vi "Main 2.vi"() -> ()   [LabVIEW 2017, in "HostCode.lvlib"]
doc: "This VI was generated automatically using the FPGA Wizard. You can modify the VI normally."
uses:
  HostCode.lvlib
  FPGACode/Lead Enum.ctl
  Trigger Params.ctl
  FPGACode/Channel Enum.ctl
  <vilib>/FPGAPlugInAG/Dynamic/niLvFpga_Reset_Dynamic.vi
  <vilib>/FPGAPlugInAG/Dynamic/niLvFpga_Run_Dynamic.vi
  <vilib>/Utility/error.llb/Error Cluster From Error Code.vi
  <vilib>/rvi/errors/niLvFpgaAdjustHostInterfaceError.vi
  <vilib>/FPGAPlugInAG/Dynamic/niLvFpga_Close_Dynamic.vi
  <vilib>/rvi/interface/nirviMethod/nirviMethod.xnode
  <vilib>/rvi/interface/nirviReadWriteControl/nirviReadWriteControl.xnode
  <vilib>/rvi/interface/nirviCloseFPGA/nirviCloseFPGA.xnode
  <vilib>/rvi/interface/Simulation/niFpgaSimulationCallBeginRW.vi
  <vilib>/FPGAPlugInAG/Dynamic/niLvFpga_ReadFifo_Dynamic.vi
  <vilib>/rvi/errors/niLvFpgaMergeErrorWithErrorCode.vi
  NiFpgaLv.dll
panel:
  in  "Beta":u8(slide)=1 scale=0.0..3.0
  in  "Sensis\nECG Scaling":i16=1 caption="ECG Output\nScaling" min=1 max=100 step=1
  in  "Tab Control":enum32{"Main", "Utilities"}(tab)
  in  "Record Only Activity":bool=TRUE
  out "ECG":i16[][](graph)
  out "Invasive Blood Pressure":i16[][](graph)=[[-20, 4166], [-20, 4166], [-20, 4165], [-20, 4165], [-19, 4165], [-19, 4165], [-18, 4163], [-18, 4165], [-18, 4166], [-18, 4166], [-18, 4166], [-18, 4165], [-18, 4165], [-18, 4164], [-18, 4164], [-18, 4165], [-19, 4166], [-20, 4166], [-20, 4164], [-20, 4164], [-20, 4165], [-20, 4165], [-19, 4165], [-19, 4164], [-18, 4165], [-18, 4166], [-18, 4165], [-18, 4166], [-18, 4165], [-18, 4165], [-18, 4165], [-18, 4165], [-19, 4165], [-20, 4165], [-20, 4165], [-20, 4165], [-20, 4166], [-20, 4167], [-20, 4166], [-19, 4164], [-18, 4163], [-18, 4164], [-18, 4165], [-18, 4166], [-17, 4165], [-18, 4166], [-18, 4166], [-18, 4165], [-18, 4166], [-19, 4165], [-20, 4164], [-20, 4165], [-20, 4166], [-20, 4166], [-20, 4167]]
  out "Trigger":i16[][](graph)
  in  "IBP Filter":bool
  in  "Plot Info":T2={"Element"={"Lead"=enum."I", "Filter"=TRUE}, "Element 2"={"Lead"=enum."II", "Filter"=TRUE}, "Element 3"={"Lead"=enum."III", "Filter"=TRUE}}
  in  "Record":bool
  in  "Path":path=path "C:/Users/IFEUser/Documents/LabVIEW Data/Saved Data/test.txt"
  out "Active":bool
  in  "Trigger 2":T3={"Channel"=enum."II", "Threshold"=1000, "d/dt"=FALSE, "Invert"=FALSE}
  in  "Invert IBP PWM":bool=TRUE
  in  "Invert ECG PWM":bool=TRUE
  in  "ECG Input\nGain":u16(ring)=1 items=["1"=1, "2"=2, "3"=3, "4"=4, "6"=0, "8"=5, "12"=6]
  in  "ECG Beta":fxp<+/-,32,-16>=1.000088900582341e-11 format="%.3e"
  in  "Filter Size":i16=100
  in  "IBP Beta":fxp<+/-,32,-16> format="%.3e"
  out "Gradients":i16[][](graph)
  in  "Offset":cluster{"X":i16, "Y":i16, "Z":i16} {"Z" format="%.2f"; "Y" format="%.2f"; "X" format="%.2f"}
  in  "High Pass Filter":bool
  out "Taps":dbl[](graph)
  out "Weights":dbl[](graph)
  out "Beta Product":fxp<+/-,32,-1> format="%.3e"
  out "Weighted Sum":fxp<+/-,33,19> format="%.3e"
  in  "Channel":i32
  in  "IBP0":T5={"Scale"=0.1669921875, "Offset"=-1795.0} {"Scale" format="%#_4g"}
  in  "IBP1":T5={"Scale"=0.169921875, "Offset"=-1935.0} {"Scale" format="%#_3g"}
  out "Loop Time":u32
  in  "Reset":bool
  in  "Start":bool
  in  "Global Stop":bool
  out "Actual Loop Rate (Ticks)":u32
  out "Late? Latched":bool
  in  "Loop Rate (Hz)":dbl=10000.0
  out "Calculated Rate (Hz)":dbl
  out "error out":errorcluster
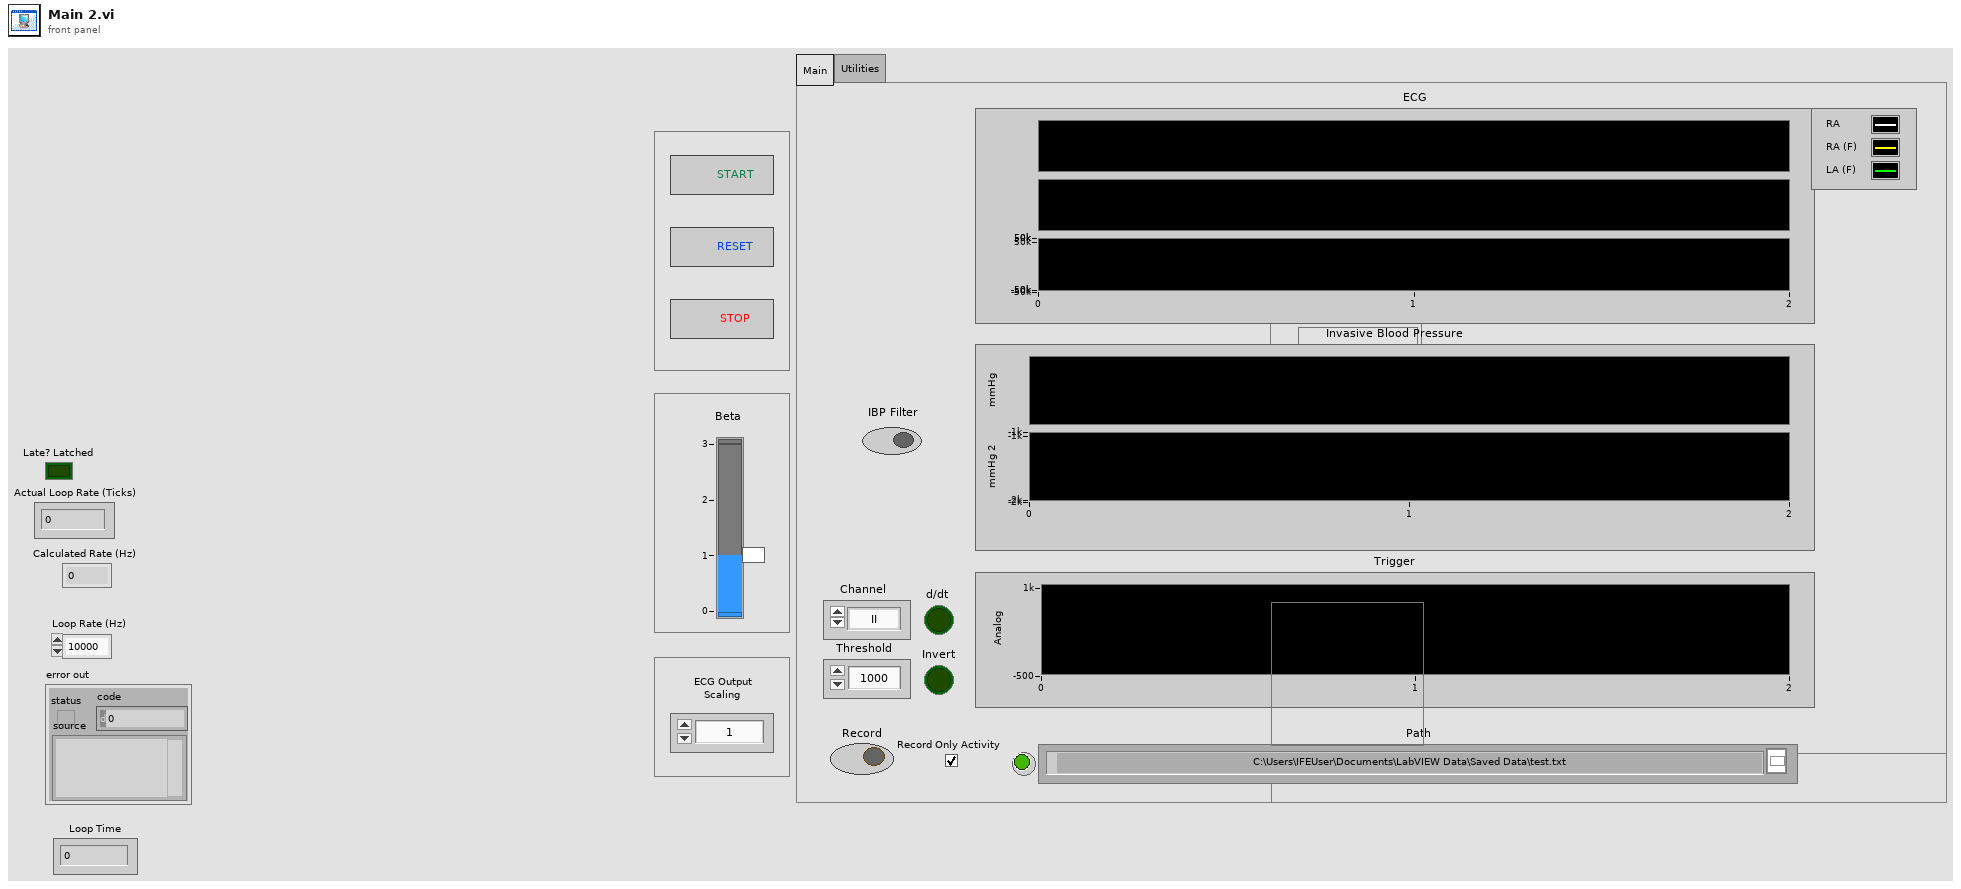
[diagram p1: front panel]
types:
  T1 = typedef "Lead Enum.ctl" = enum16{"RA", "LA", "LL", "V1", "V2", "V3", "V4", "V5", "V6", "I", "II", "III", "aVR", "aVL", "aVF", "Vw"}
  T2 = cluster{"Element":cluster{"Lead":T1, "Filter":bool}, "Element 2":cluster{"Lead":T1, "Filter":bool}, "Element 3":cluster{"Lead":T1, "Filter":bool}}
  T3 = typedef "Trigger Params.ctl" = cluster{"Channel":T4, "Threshold":i16, "d/dt":bool, "Invert":bool}
  T4 = typedef "Channel Enum.ctl" = enum16{"RA", "LA", "LL", "V1", "V2", "V3", "V4", "V5", "V6", "I", "II", "III", "aVR", "aVL", "aVF", "Vw", "IBP1", "IBP2"}
  T5 = cluster{"Scale":fxp<+/-,16,5>, "Offset":fxp<+/-,16,16>}
  T6 = enum32{"invalid app kind", "Development System", "Run Time System", "Student Edition", "Embedded LabVIEW", "Evaluation", "Custom"}
  T7 = enum8{"Enabled", "Disabled", "Disabled and Grayed Out"}
  T8 = typedef "LVOffsetAndMultiplierTypeDef.ctl" = cluster{"Offset":dbl, "Multiplier":dbl}
  T9 = enum16{"open", "replace", "create", "open or create", "replace or create", "replace or create with confirmation"}
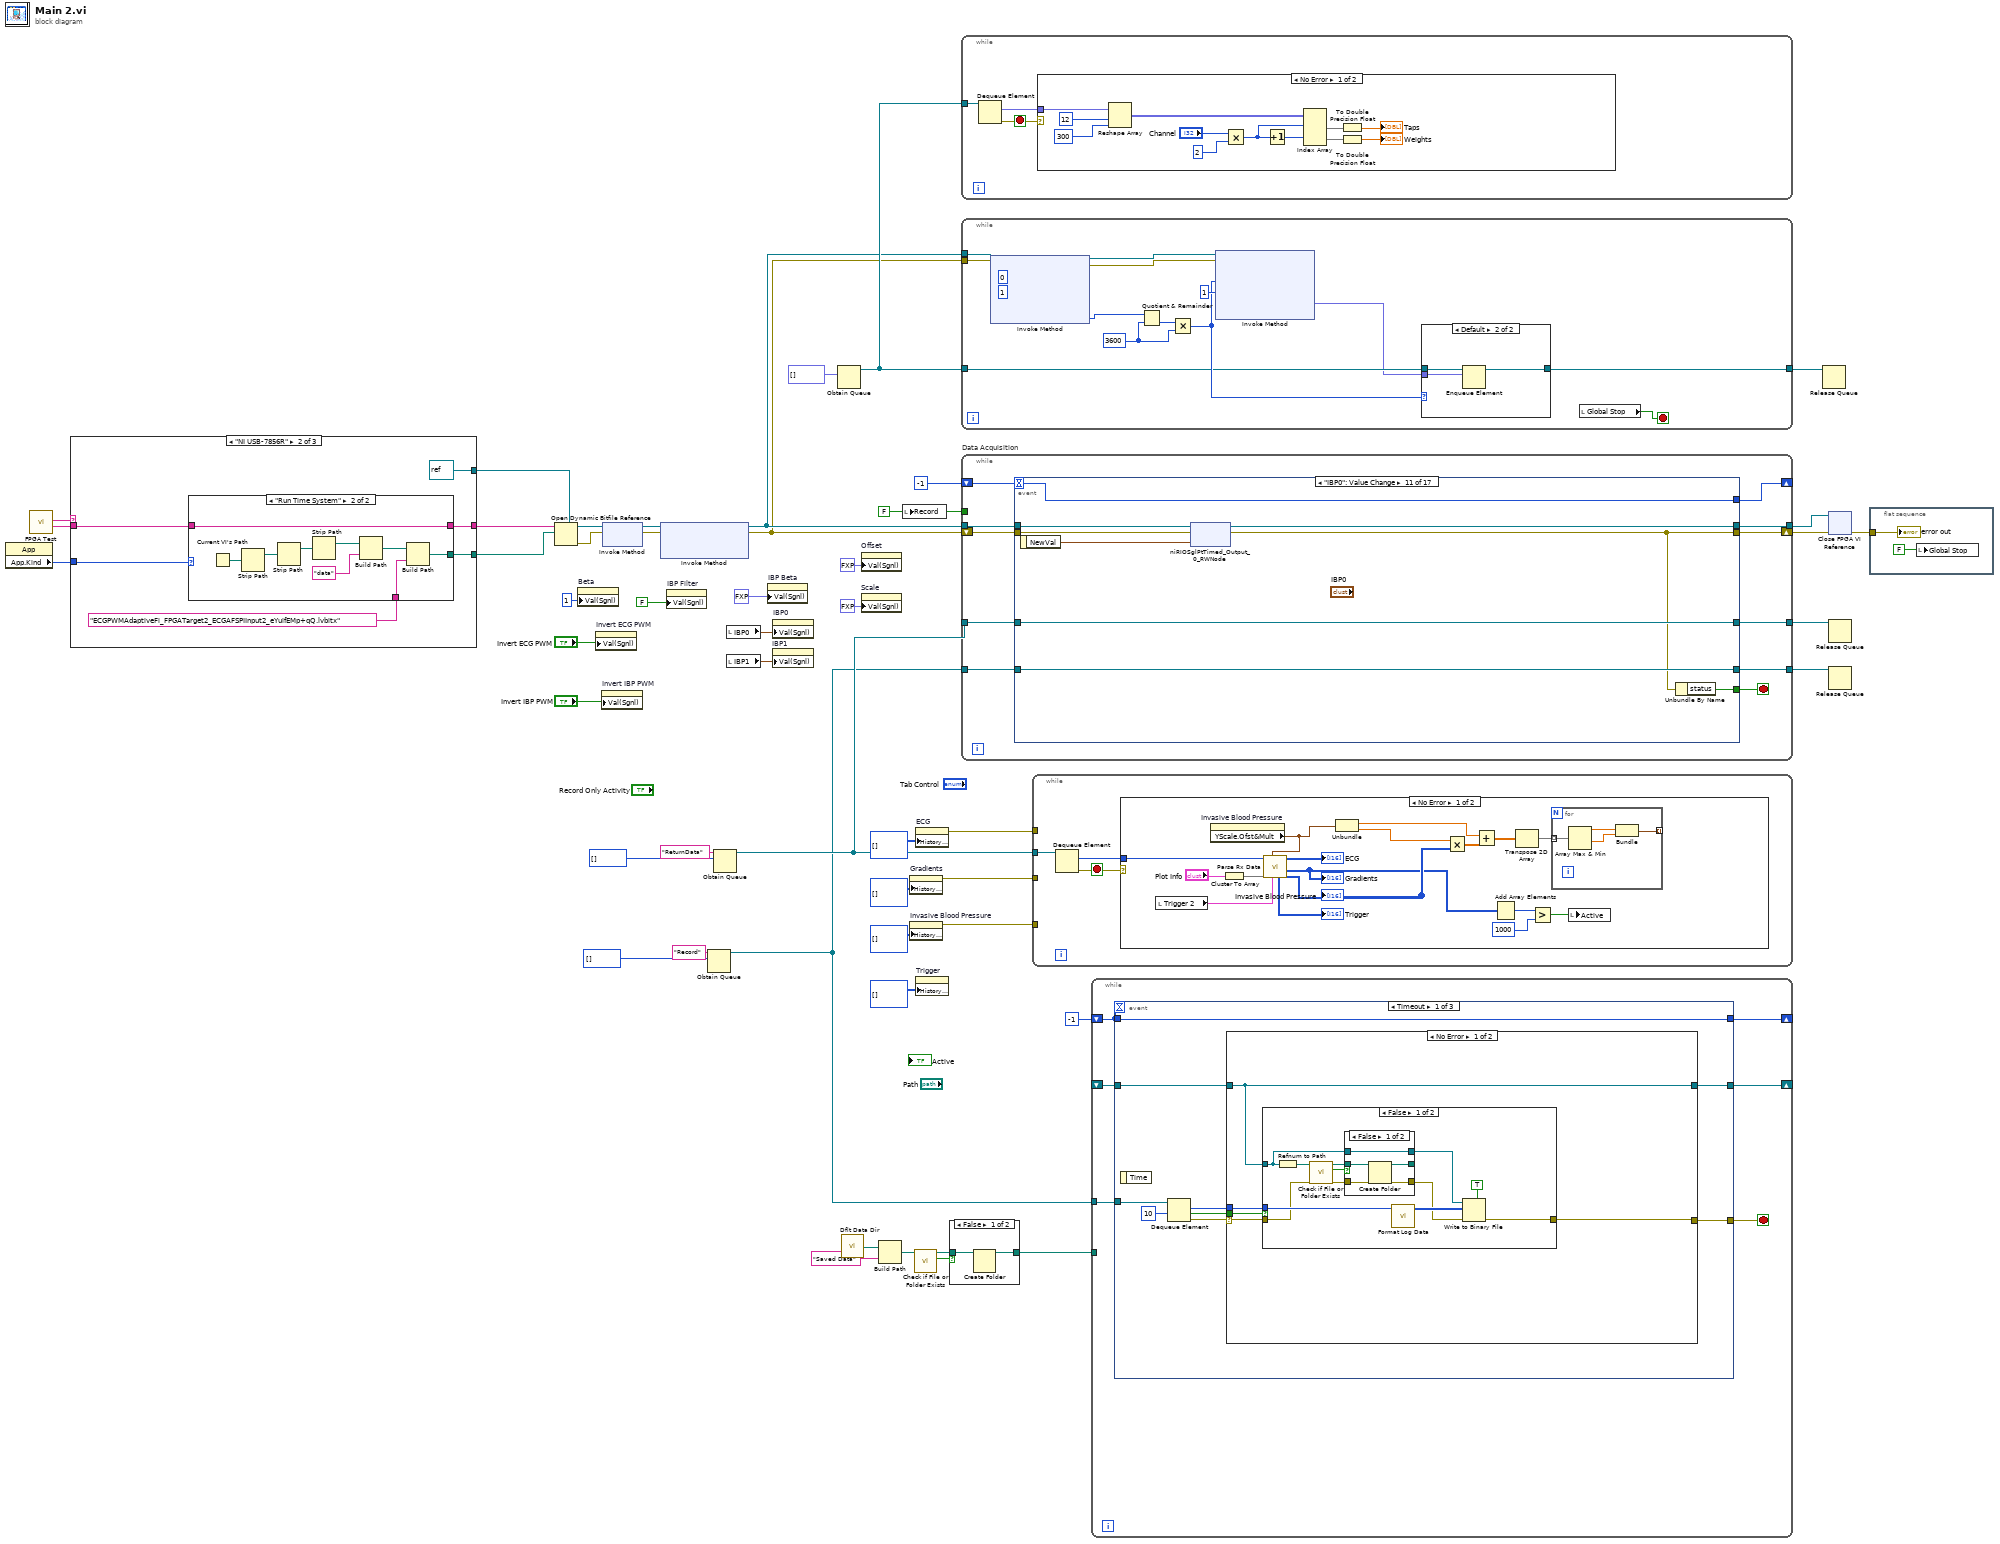
[diagram p0: block diagram]
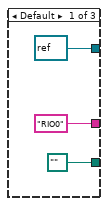
[diagram p3: hidden frame]
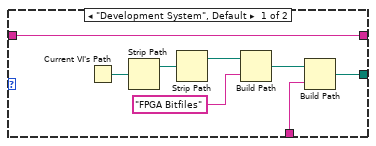
[diagram p4: hidden frame]
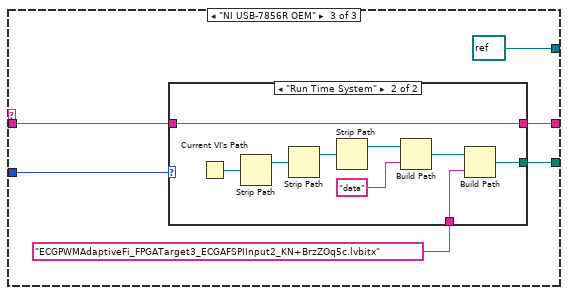
[diagram p5: hidden frame]
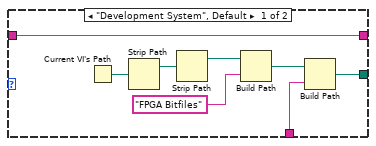
[diagram p6: hidden frame]
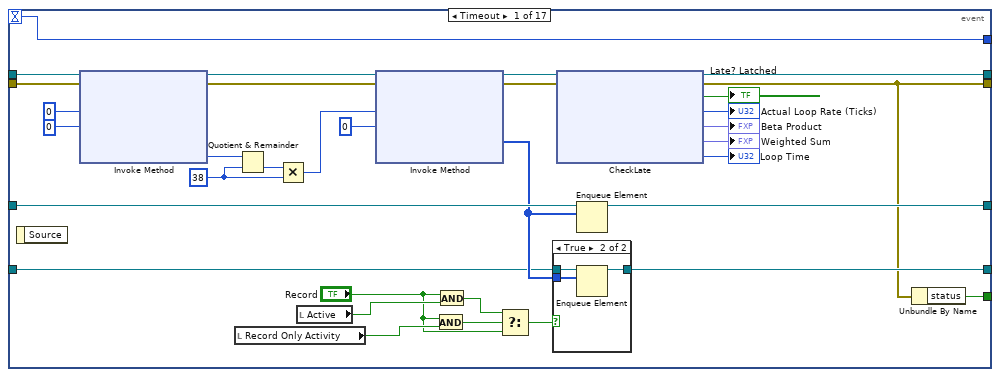
[diagram p7: hidden frame]
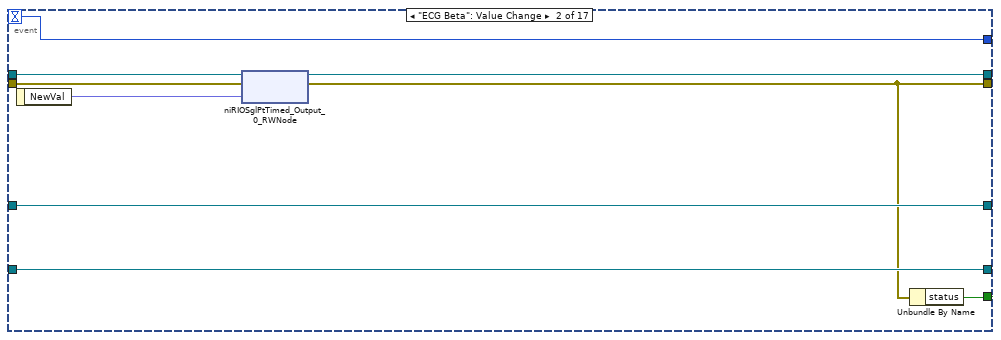
[diagram p9: hidden frame]
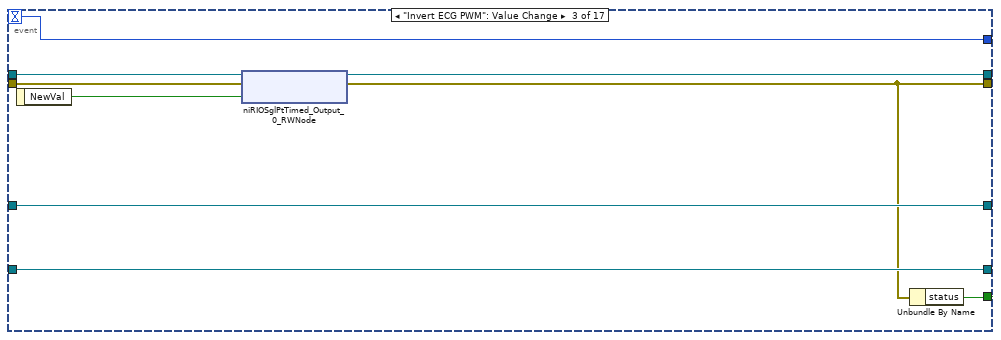
[diagram p10: hidden frame]
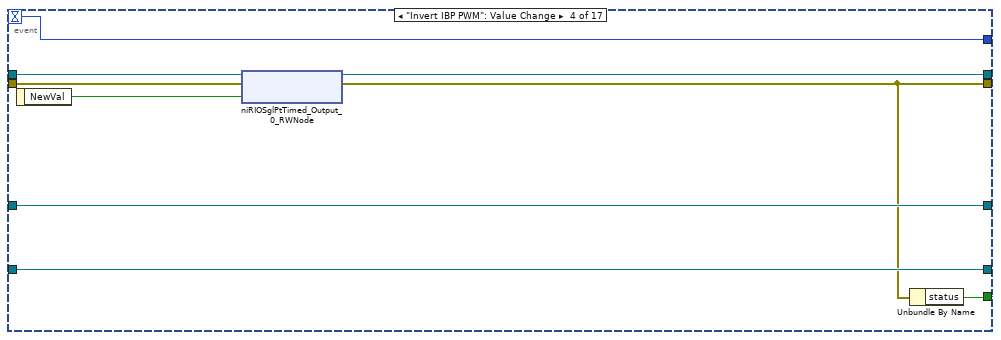
[diagram p11: hidden frame]
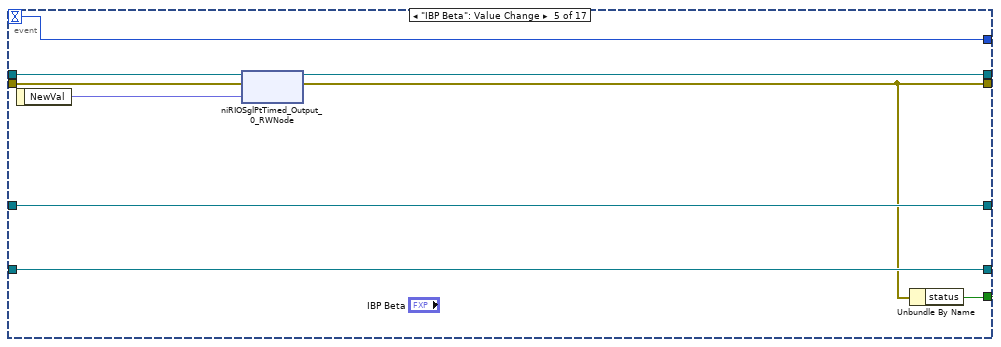
[diagram p12: hidden frame]
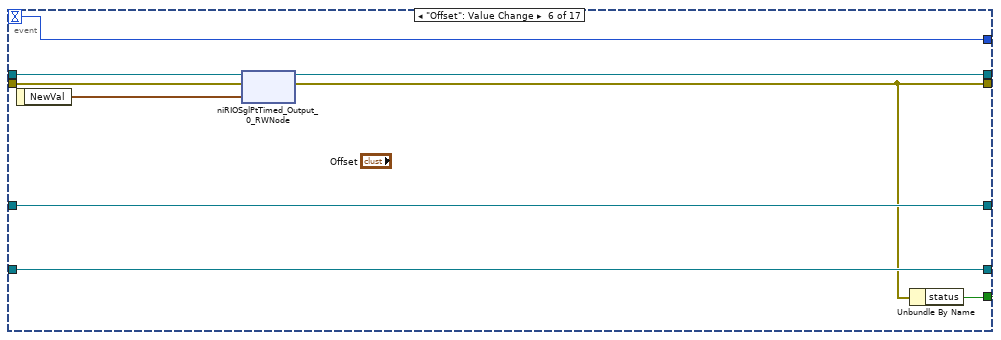
[diagram p13: hidden frame]
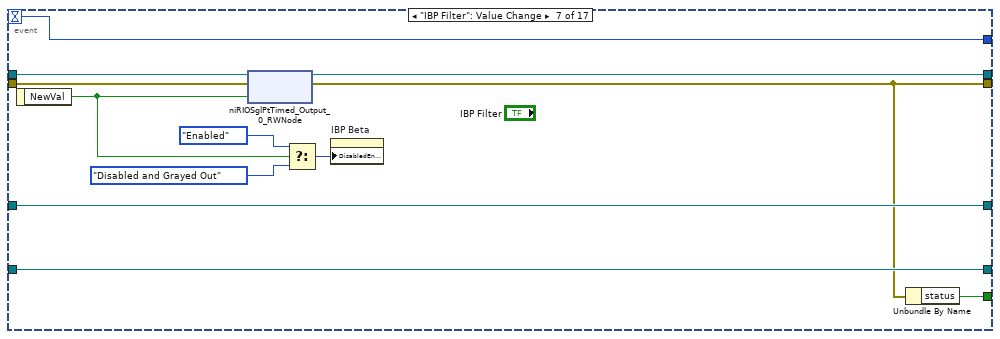
[diagram p14: hidden frame]
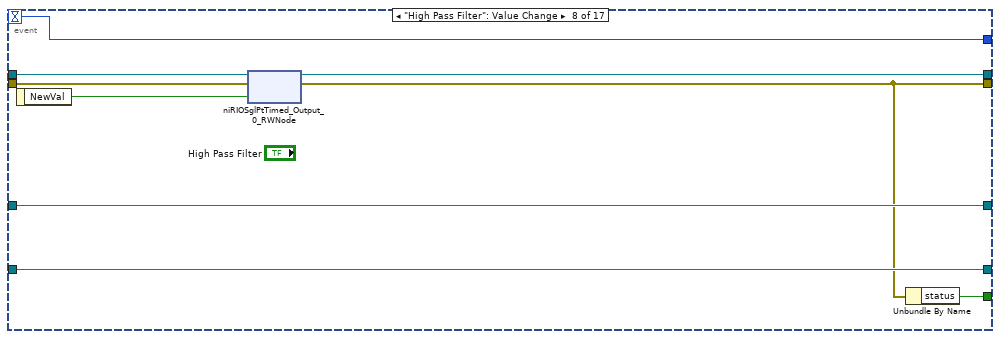
[diagram p15: hidden frame]
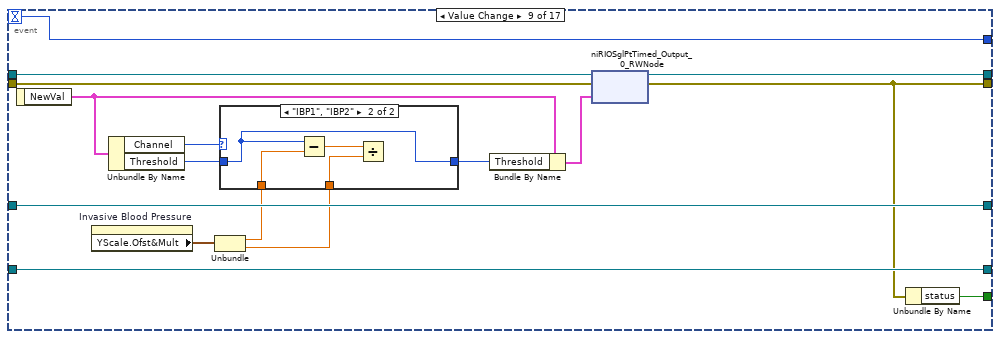
[diagram p16: hidden frame]
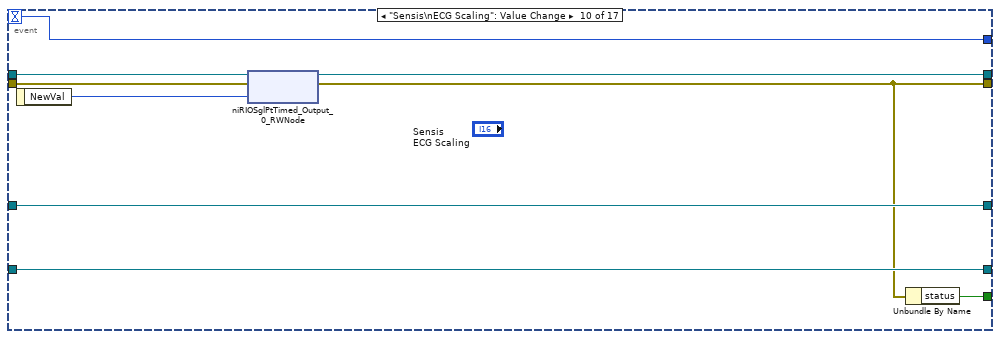
[diagram p18: hidden frame]
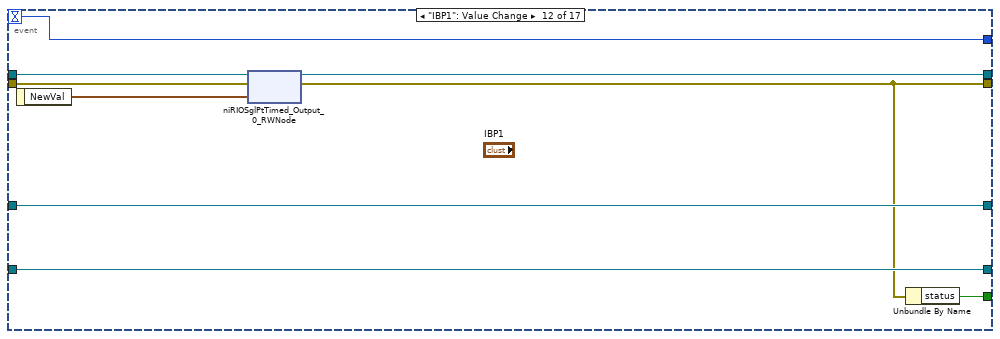
[diagram p19: hidden frame]
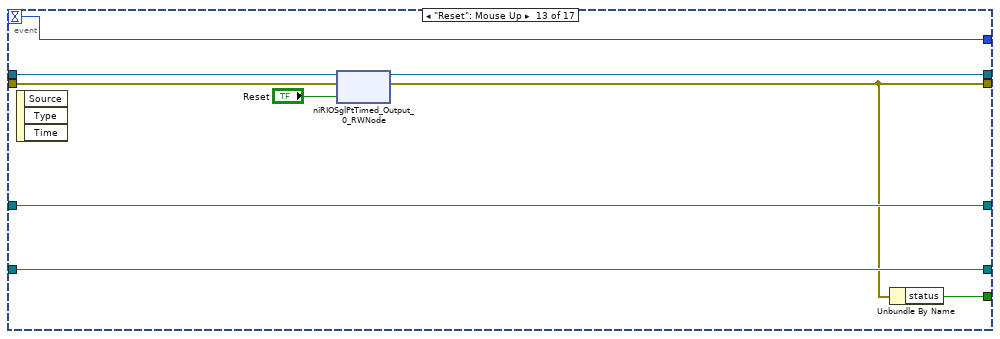
[diagram p20: hidden frame]
diagram:
  w2 = FALSE ("Record")
  n1 = property class="App"() -> ("App.Kind"=w13:T6)  [unwired: 2 in, 2 out]
  n2 = call "FPGA Test.vi"() -> ("Resource"=w12:string, "ProdName"=w11:string)  [unwired: 10 in]
  n3 = case shown="\"NI USB-7856R\"" w11 {
    tunnel: [path "" ("appended path") w60 w83] -> w14
    tunnel: w13 -> [_ w59 w82]
    tunnel: w12 -> [_ w58 w81]
    tunnel: ["RIO0" ("Device address") w56 w79] -> w10
    tunnel: [refnum<k20> refnum ("FPGA Interface") refnum<k20> refnum ("FPGA Interface") refnum<k20> refnum ("FPGA Interface")] -> w1
    frame Default {
    }
    frame "NI USB-7856R" {
      n4 = case shown="\"Run Time System\"" w59 {
        tunnel: [w63 w72] -> w60
        tunnel: w58 -> [w61 w69]
        tunnel: "ECGPWMAdaptiveFi_FPGATarget2_ECGAFSPIInput2_eYuifEMp+qQ.lvbitx" ("name or relative path") -> [w62 w70]
        tunnel: [w61 w69] -> w56
        frame "Development System", Default {
          n5 = Current VI's Path() -> (path=w68:path)
          n6 = Strip Path(path=w68) -> (stripped path=w65:path)  [unwired: 1 out]
          n7 = Strip Path(path=w65) -> (stripped path=w64:path)  [unwired: 1 out]
          n8 = Build Path(base path=w64, name or relative path="FPGA Bitfiles") -> (appended path=w66:path)
          n9 = Build Path(base path=w66, name or relative path=w62) -> (appended path=w63:path)
        }
        frame "Run Time System" {
          n10 = Current VI's Path() -> (path=w77:path)
          n11 = Strip Path(path=w77) -> (stripped path=w74:path)  [unwired: 1 out]
          n12 = Strip Path(path=w74) -> (stripped path=w73:path)  [unwired: 1 out]
          n13 = Strip Path(path=w73) -> (stripped path=w71:path)  [unwired: 1 out]
          n14 = Build Path(base path=w71, name or relative path="data") -> (appended path=w75:path)
          n15 = Build Path(base path=w75, name or relative path=w70) -> (appended path=w72:path)
        }
      }
    }
    frame "NI USB-7856R OEM" {
      n16 = case shown="\"Run Time System\"" w82 {
        tunnel: [w86 w95] -> w83
        tunnel: w81 -> [w84 w92]
        tunnel: "ECGPWMAdaptiveFi_FPGATarget3_ECGAFSPIInput2_KN+BrzZOq5c.lvbitx" ("name or relative path") -> [w85 w93]
        tunnel: [w84 w92] -> w79
        frame "Development System", Default {
          n17 = Current VI's Path() -> (path=w91:path)
          n18 = Strip Path(path=w91) -> (stripped path=w88:path)  [unwired: 1 out]
          n19 = Strip Path(path=w88) -> (stripped path=w87:path)  [unwired: 1 out]
          n20 = Build Path(base path=w87, name or relative path="FPGA Bitfiles") -> (appended path=w89:path)
          n21 = Build Path(base path=w89, name or relative path=w85) -> (appended path=w86:path)
        }
        frame "Run Time System" {
          n22 = Current VI's Path() -> (path=w100:path)
          n23 = Strip Path(path=w100) -> (stripped path=w97:path)  [unwired: 1 out]
          n24 = Strip Path(path=w97) -> (stripped path=w96:path)  [unwired: 1 out]
          n25 = Strip Path(path=w96) -> (stripped path=w94:path)  [unwired: 1 out]
          n26 = Build Path(base path=w94, name or relative path="data") -> (appended path=w98:path)
          n27 = Build Path(base path=w98, name or relative path=w93) -> (appended path=w95:path)
        }
      }
    }
  }
  n28 = Open Dynamic Bitfile Reference(0:w10, 1:w14, 4:w1) -> (5:w16:refnum<k20>, 8:w15:errorcluster)  [unwired: 2 in]
  n29 = property on="Beta" class="Slide (strict)"("Val(Sgnl)"=u8 1 ("Value (Signaling)")) -> ()  [unwired: 2 in, 2 out]
  n30 = property on="Invert ECG PWM" class="Bool (strict)"("Val(Sgnl)"="Invert ECG PWM") -> ()  [unwired: 2 in, 2 out]
  n31 = property on="Invert IBP PWM" class="Bool (strict)"("Val(Sgnl)"="Invert IBP PWM") -> ()  [unwired: 2 in, 2 out]
  n32 = xnode ("Invoke Method")("FPGA VI Reference In"=w16, "error in"=w15) -> ("FPGA VI Reference Out"=w30:refnum<k20>, "error out"=w51:errorcluster)
  n33 = xnode ("Invoke Method")("FPGA VI Reference In"=w30, "error in"=w51) -> ("FPGA VI Reference Out"=w28:refnum<k20>, "error out"=w27:errorcluster)  [unwired: 1 in]
  n34 = property on="IBP Filter" class="Bool (strict)"("Val(Sgnl)"=FALSE ("Value (Signaling)")) -> ()  [unwired: 2 in, 2 out]
  n35 = Obtain Queue(name (unnamed)="Record", element data type=i16[] []) -> (queue out=w37:refnum<queue>)  [unwired: 3 in, 2 out]
  n36 = Obtain Queue(name (unnamed)="ReturnData", element data type=i16[] []) -> (queue out=w45:refnum<queue>)  [unwired: 3 in, 2 out]
  n37 = local read "IBP0"() -> (w20:T5)
  n38 = local read "IBP1"() -> (w19:T5)
  n39 = property on="IBP Beta" class="DigNum (strict)"("Val(Sgnl)"=fxp<+/-,32,-16> 0.0 ("Value (Signaling)")) -> ()  [unwired: 2 in, 2 out]
  n40 = property on="IBP0" class="Clust (strict)"("Val(Sgnl)"=w20) -> ()  [unwired: 2 in, 2 out]
  n41 = property on="IBP1" class="Clust (strict)"("Val(Sgnl)"=w19) -> ()  [unwired: 2 in, 2 out]
  n42 = Obtain Queue(element data type=fxp<+/-,32,16>[] [] ("Data")) -> (queue out=w33:refnum<queue>)  [unwired: 4 in, 2 out]
  n43 = call <vilib>:"Dflt Data Dir.vi"() -> ("App:Default Data Directory"=w9:path)
  n44 = property on="Offset" class="DigNum (strict)"("Val(Sgnl)"=fxp<+/-,16,16> 0.0 ("Value (Signaling)")) -> ()  [unwired: 2 in, 2 out]
  n45 = property on="Scale" class="DigNum (strict)"("Val(Sgnl)"=fxp<+/-,16,5> 1.0 ("Value (Signaling)")) -> ()  [unwired: 2 in, 2 out]
  n46 = Build Path(base path=w9, name or relative path="Saved Data") -> (appended path=w7:path)
  n47 = local write "Record"(w2) -> ()
  n48 = property on="Gradients" class="WFChart (strict)"("History Data"=i16[][] []) -> (error out=w42:errorcluster)  [unwired: 2 in, 1 out]
  n49 = property on="Invasive Blood Pressure" class="WFChart (strict)"("History Data"=i16[][] []) -> (error out=w34:errorcluster)  [unwired: 2 in, 1 out]
  n50 = call <vilib>:"Check if File or Folder Exists.vi"("path"=w7) -> ("file or folder exists?"=w6:bool, "dup path"=w5:path)  [unwired: 8 in, 1 out]
  n51 = property on="ECG" class="WFChart (strict)"("History Data"=i16[][] []) -> (error out=w43:errorcluster)  [unwired: 2 in, 1 out]
  n52 = property on="Trigger" class="WFChart (strict)"("History Data"=i16[][] []) -> ()  [unwired: 2 in, 2 out]
  n53 = case shown="False" w6 {
    tunnel: w5 -> [w102 w103]
    tunnel: [w101 w103] -> w3
    frame False {
      n54 = Create Folder(path (use dialog)=w102) -> (created path=w101:path)  [unwired: 2 in, 2 out]
    }
    frame True {
    }
  }
  n55 = while {
    tunnel: w33 -> [w106]
    stop <- w104 stop-if-true
    n56 = Dequeue Element(queue=w106) -> (element=w105:fxp<+/-,32,16>[], error out=w104:errorcluster)  [unwired: 2 in, 2 out]
    n57 = case shown="No Error" w104 {
      tunnel: w105 -> [w118 _]
      frame No Error {
        n58 = Reshape Array(w118, 12 ("dimension size"), 300 ("dimension size")) -> (w114:fxp<+/-,32,16>[][])
        n59 = Multiply(x="Channel", y=2) -> (x*y=w107:i32)
        n60 = Increment(x=w107) -> (x+1=w108:i32)
        n61 = Index Array(array=w114, index (row) #1=w107, index (row) #2=w108) -> (element #1=w113:fxp<+/-,32,16>[], element #2=w112:fxp<+/-,32,16>[])  [unwired: 2 in]
        n62 = To Double Precision Float(number=w113) -> (double precision float=→"Taps":dbl[])
        n63 = To Double Precision Float(number=w112) -> (double precision float=→"Weights":dbl[])
      }
      frame Error {
      }
    }
  }
  n64 = while {
    tunnel: w28 -> [w133]
    tunnel: w27 -> [w132]
    tunnel: w33 -> [w121]
    tunnel: [w119] -> w32
    stop <- w124 stop-if-true
    w126 = u32 3600 ("y")
    n65 = xnode "Invoke Method"("FPGA VI Reference In"=w133, "error in"=w132, "Number of Elements"=u32 0, "Timeout (ms)"=1) -> ("FPGA VI Reference Out"=w129:refnum<k20>, "error out"=w128:errorcluster, "Elements Remaining"=w125:u32)  [unwired: 1 out]
    n66 = Quotient & Remainder(x=w125, y=w126) -> (floor(x/y)=w127:u32)  [unwired: 1 out]
    n67 = Multiply(x=w127, y=w126) -> (x*y=w122:u32)
    n68 = xnode "Invoke Method"("FPGA VI Reference In"=w129, "error in"=w128, "Number of Elements"=w122, "Timeout (ms)"=1) -> ("Data"=w120:fxp<+/-,32,16>[])  [unwired: 3 out]
    n69 = case shown="Default" w122 {
      tunnel: w121 -> [w134 w137]
      tunnel: w120 -> [_ w136]
      tunnel: [w134 w135] -> w119
      frame 0 {
      }
      frame Default {
        n70 = Enqueue Element(queue=w137, element=w136) -> (queue out=w135:refnum<queue>)  [unwired: 2 in, 2 out]
      }
    }
    n71 = local read "Global Stop"() -> (w124:bool)
  }
  n72 = while "Data Acquisition" {
    tunnel: w28 -> [w144]
    shift-right: [w148] -> w50
    shift-left: w27 -> [w145]
    tunnel: [w146] -> w48
    tunnel: w45 -> [w143]
    tunnel: [w142] -> w40
    tunnel: w37 -> [w141]
    tunnel: [w140] -> w36
    shift-right: [w138] -> _
    shift-left: -1 -> [w139]
    tunnel: w2 -> [_]
    stop <- w147 stop-if-true
    n73 = event shown="[10] \"IBP0\": Value Change" {
      selector: _ -> [_ _ _ _ _ _ _ _ _ _ _ _ _ _ _ _ _]
      dyn-events: _ -> [_ _ _ _ _ _ _ _ _ _ _ _ _ _ _ _ _]
      timeout: w139 -> [w157 w188 w197 w206 w215 w224 w237 w245 w262 w276 w285 w294 w302 _ w331 w342 w351]
      tunnel: [w156 w187 w196 w205 w214 w223 w236 w244 w261 w275 w284 w293 w301 w312 w332 w343 w350] -> w148
      tunnel: [w155 w186 w195 w204 w213 w222 w235 w243 w260 w274 w283 w292 w300 w311 TRUE FALSE ("status") FALSE ("status")] -> w147
      tunnel: [w181 w192 w201 w210 w219 w228 w240 w249 w265 w279 w288 w297 w306 w316 w333 w344 w352] -> w146
      tunnel: w145 -> [w159 w193 w202 w211 w220 w229 w241 w250 w266 w280 w289 w298 w307 w326 w334 w343 w350]
      tunnel: w144 -> [w160 w194 w203 w212 w221 w230 w242 w251 w267 w281 w290 w299 w308 w327 w335 w344 w352]
      tunnel: w143 -> [w170 w190 w199 w208 w217 w226 w239 w247 w264 w278 w287 w296 w305 w325 w338 w341 w349]
      tunnel: [w166 w190 w199 w208 w217 w226 w239 w247 w264 w278 w287 w296 w305 w325 w338 w341 w349] -> w142
      tunnel: w141 -> [w164 w189 w198 w207 w216 w225 w238 w246 w263 w277 w286 w295 w304 w324 w337 w340 w348]
      tunnel: [w158 w189 w198 w207 w216 w225 w238 w246 w263 w277 w286 w295 w304 w324 w337 w340 w348] -> w140
      tunnel: [w157 w188 w197 w206 w215 w224 w237 w245 w262 w276 w285 w294 w302 50 w331 w342 w351] -> w138
      event Timeout {
        w168 = u32 38 ("y")
        n74 = event-data() -> ()  [unwired: 1 in, 1 out]
        n75 = xnode "Invoke Method"("FPGA VI Reference In"=w160, "error in"=w159, "Number of Elements"=u32 0, "Timeout (ms)"=0) -> ("FPGA VI Reference Out"=w176:refnum<k20>, "error out"=w175:errorcluster, "Elements Remaining"=w174:u32)  [unwired: 1 out]
        n76 = local read "Record Only Activity"() -> (w151:bool)
        n77 = Quotient & Remainder(x=w174, y=w168) -> (floor(x/y)=w169:u32)  [unwired: 1 out]
        n78 = Multiply(x=w169, y=w168) -> (x*y=w167:u32)
        n79 = local read "Active"() -> (w154:bool)
        n80 = xnode "Invoke Method"("FPGA VI Reference In"=w176, "error in"=w175, "Number of Elements"=w167, "Timeout (ms)"=0) -> ("FPGA VI Reference Out"=w172:refnum<k20>, "error out"=w171:errorcluster, "Data"=w165:i16[])  [unwired: 1 out]
        n81 = And(x="Record", y=w151) -> (x .and. y?=w150:bool)
        n82 = And(x="Record", y=w154) -> (x .and. y?=w153:bool)
        n83 = Select(t=w153, s=w150, f="Record") -> (s? t:f=w152:bool)
        n84 = case shown="True" w152 {
          tunnel: w165 -> [_ w185]
          tunnel: w164 -> [w182 w184]
          tunnel: [w182 w183] -> w158
          frame False {
          }
          frame True {
            n85 = Enqueue Element(queue=w184, element=w185) -> (queue out=w183:refnum<queue>)  [unwired: 2 in, 2 out]
          }
        }
        n86 = xnode ("CheckLate")("FPGA VI Reference In"=w172, "error in"=w171) -> ("FPGA VI Reference Out"=w181:refnum<k20>, "error out"=w156:errorcluster, "Late? Latched"=→"Late? Latched":bool, "Actual Loop Rate (Ticks)"=→"Actual Loop Rate (Ticks)":u32, "BetaProduct"=→"Beta Product":fxp<+/-,32,-1>, "WeightSum"=→"Weighted Sum":fxp<+/-,33,19>, "Loop Time"=→"Loop Time":u32)
        n87 = Enqueue Element(queue=w170, element=w165) -> (queue out=w166:refnum<queue>)  [unwired: 2 in, 2 out]
        n88 = Unbundle By Name(w156) -> ("status"=w155:bool)
      }
      event "ECG Beta": Value Change {
        n89 = event-data() -> ("NewVal"=w191:fxp<+/-,32,-16>)  [unwired: 1 in]
        n90 = xnode ("niRIOSglPtTimed_Output_0_RWNode")("FPGA VI Reference In"=w194, "error in"=w193, "Beta ECG"=w191) -> ("FPGA VI Reference Out"=w192:refnum<k20>, "error out"=w187:errorcluster)
        n91 = Unbundle By Name(w187) -> ("status"=w186:bool)
      }
      event "Invert ECG PWM": Value Change {
        n92 = event-data() -> ("NewVal"=w200:bool)  [unwired: 1 in]
        n93 = xnode ("niRIOSglPtTimed_Output_0_RWNode")("FPGA VI Reference In"=w203, "error in"=w202, "Invert PWM ECG"=w200) -> ("FPGA VI Reference Out"=w201:refnum<k20>, "error out"=w196:errorcluster)
        n94 = Unbundle By Name(w196) -> ("status"=w195:bool)
      }
      event "Invert IBP PWM": Value Change {
        n95 = event-data() -> ("NewVal"=w209:bool)  [unwired: 1 in]
        n96 = xnode ("niRIOSglPtTimed_Output_0_RWNode")("FPGA VI Reference In"=w212, "error in"=w211, "Invert PWM IBP"=w209) -> ("FPGA VI Reference Out"=w210:refnum<k20>, "error out"=w205:errorcluster)
        n97 = Unbundle By Name(w205) -> ("status"=w204:bool)
      }
      event "IBP Beta": Value Change {
        n98 = event-data() -> ("NewVal"=w218:fxp<+/-,32,-16>)  [unwired: 1 in]
        n99 = xnode ("niRIOSglPtTimed_Output_0_RWNode")("FPGA VI Reference In"=w221, "error in"=w220, "Beta IBP"=w218) -> ("FPGA VI Reference Out"=w219:refnum<k20>, "error out"=w214:errorcluster)
        n100 = Unbundle By Name(w214) -> ("status"=w213:bool)
      }
      event "Offset": Value Change {
        n101 = event-data() -> ("NewVal"=w227:cluster{"X":i16, "Y":i16, "Z":i16})  [unwired: 1 in]
        n102 = xnode ("niRIOSglPtTimed_Output_0_RWNode")("FPGA VI Reference In"=w230, "error in"=w229, "Offset"=w227) -> ("FPGA VI Reference Out"=w228:refnum<k20>, "error out"=w223:errorcluster)
        n103 = Unbundle By Name(w223) -> ("status"=w222:bool)
      }
      event "IBP Filter": Value Change {
        n104 = event-data() -> ("NewVal"=w234:bool)  [unwired: 1 in]
        n105 = xnode ("niRIOSglPtTimed_Output_0_RWNode")("FPGA VI Reference In"=w242, "error in"=w241, "IBP Filter"=w234) -> ("FPGA VI Reference Out"=w240:refnum<k20>, "error out"=w236:errorcluster)
        n106 = Select(t=T7."Enabled" ("Disabled"), s=w234, f=T7."Disabled and Grayed Out" ("Disabled")) -> (s? t:f=w231:T7)
        n107 = property on="IBP Beta" class="DigNum (strict)"("DisabledEnum"=w231) -> ()  [unwired: 2 in, 2 out]
        n108 = Unbundle By Name(w236) -> ("status"=w235:bool)
      }
      event "High Pass Filter": Value Change {
        n109 = event-data() -> ("NewVal"=w248:bool)  [unwired: 1 in]
        n110 = xnode ("niRIOSglPtTimed_Output_0_RWNode")("FPGA VI Reference In"=w251, "error in"=w250, "HPF"=w248) -> ("FPGA VI Reference Out"=w249:refnum<k20>, "error out"=w244:errorcluster)
        n111 = Unbundle By Name(w244) -> ("status"=w243:bool)
      }
      event Value Change {
        n112 = event-data() -> ("NewVal"=w257:T3)  [unwired: 1 in]
        n113 = property on="Invasive Blood Pressure" class="WFChart (strict)"() -> ("YScale.Ofst&Mult"=w254:T8)  [unwired: 2 in, 2 out]
        n114 = Unbundle By Name(w257) -> ("Channel"=w259:T4, "Threshold"=w258:i16)
        n115 = Unbundle(w254) -> ("Offset"=w253:dbl, "Multiplier"=w252:dbl)
        n116 = case shown="\"IBP1\", \"IBP2\"" w259 {
          tunnel: w258 -> [w268 w269]
          tunnel: [w268 w269] -> w256
          tunnel: w253 -> [_ w272]
          tunnel: w252 -> [_ w270]
          frame Default {
          }
          frame "IBP1", "IBP2" {
            n117 = Subtract(x=w269, y=w272) -> (x-y=w271:dbl)
            n118 = Divide(x=w271, y=w270) -> ()  [unwired: 1 out]
          }
        }
        n119 = Bundle By Name(cluster=w257, "Threshold"=w256) -> (w255:T3)
        n120 = xnode ("niRIOSglPtTimed_Output_0_RWNode")("FPGA VI Reference In"=w267, "error in"=w266, "Trigger"=w255) -> ("FPGA VI Reference Out"=w265:refnum<k20>, "error out"=w261:errorcluster)
        n121 = Unbundle By Name(w261) -> ("status"=w260:bool)
      }
      event "Sensis\nECG Scaling": Value Change {
        n122 = event-data() -> ("NewVal"=w273:i16)  [unwired: 1 in]
        n123 = xnode ("niRIOSglPtTimed_Output_0_RWNode")("FPGA VI Reference In"=w281, "error in"=w280, "ECG Scale"=w273) -> ("FPGA VI Reference Out"=w279:refnum<k20>, "error out"=w275:errorcluster)
        n124 = Unbundle By Name(w275) -> ("status"=w274:bool)
      }
      event "IBP0": Value Change {
        n125 = event-data() -> ("NewVal"=w282:T5)  [unwired: 1 in]
        n126 = xnode ("niRIOSglPtTimed_Output_0_RWNode")("FPGA VI Reference In"=w290, "error in"=w289, "IBP0"=w282) -> ("FPGA VI Reference Out"=w288:refnum<k20>, "error out"=w284:errorcluster)
        n127 = Unbundle By Name(w284) -> ("status"=w283:bool)
      }
      event "IBP1": Value Change {
        n128 = event-data() -> ("NewVal"=w291:T5)  [unwired: 1 in]
        n129 = xnode ("niRIOSglPtTimed_Output_0_RWNode")("FPGA VI Reference In"=w299, "error in"=w298, "IBP1"=w291) -> ("FPGA VI Reference Out"=w297:refnum<k20>, "error out"=w293:errorcluster)
        n130 = Unbundle By Name(w293) -> ("status"=w292:bool)
      }
      event "Reset": Mouse Up {
        n131 = event-data() -> ()  [unwired: 1 in, 3 out]
        n132 = xnode ("niRIOSglPtTimed_Output_0_RWNode")("FPGA VI Reference In"=w308, "error in"=w307, "Reset"="Reset") -> ("FPGA VI Reference Out"=w306:refnum<k20>, "error out"=w301:errorcluster)
        n133 = Unbundle By Name(w301) -> ("status"=w300:bool)
      }
      event "Start": Mouse Up {
        w323 = 40000000.0  # FPGA Top-Level Clock Frequency
        n134 = event-data() -> ()  [unwired: 1 in, 1 out]
        n135 = call "FrequencyCoercion.vi"("Loop Rate (Hz)"="Loop Rate (Hz)", "FPGA Top-Level Clock Frequency"=w323) -> ("Actual Rate (Hz)"=→"Calculated Rate (Hz)":dbl, "FPGA Ticks"=w320:u32)  [unwired: 2 in]
        n136 = local read "Sensis\nECG Scaling"() -> (w309:i16)
        n137 = xnode ("LoopStart")("FPGA VI Reference In"=w327, "error in"=w326, "Loop Rate (Ticks)"=w320, "Filter Size"="Filter Size", "ECG Scale"=w309) -> ("FPGA VI Reference Out"=w318:refnum<k20>, "error out"=w317:errorcluster)
        n138 = property on="ECG Beta" class="DigNum (strict)"("Val(Sgnl)"="ECG Beta") -> ()  [unwired: 2 in, 2 out]
        n139 = xnode ("LoopStart")("FPGA VI Reference In"=w318, "error in"=w317, "Start"=TRUE ("Start 0"), "Start"=FALSE ("Start 0")) -> ("FPGA VI Reference Out"=w316:refnum<k20>, "error out"=w312:errorcluster)
        n140 = property on="Trigger 2" class="Clust (strict)"("Val(Sgnl)"="Trigger 2") -> ()  [unwired: 2 in, 2 out]
        n141 = Unbundle By Name(w312) -> ("status"=w311:bool)
      }
      event "Global Stop": Mouse Up {
        n142 = event-data() -> ()  [unwired: 1 in, 1 out]
        n143 = xnode ("LoopStart")("FPGA VI Reference In"=w335, "error in"=w334, "Stop"=TRUE ("stop"), "Stop"=FALSE ("stop")) -> ("FPGA VI Reference Out"=w333:refnum<k20>, "error out"=w332:errorcluster)
      }
      event "ECG Input\nGain": Value Change {
        n144 = event-data() -> ()  [unwired: 1 in, 1 out]
      }
      event "Beta": Value Change {
        n145 = event-data() -> ("NewVal"=w346:u8)  [unwired: 1 in]
        n146 = case shown="0, Default" w346 {
          tunnel: [fxp<+/-,32,-16> 0.0 ("Value (Signaling)") fxp<+/-,32,-16> 1.000088900582341e-11 ("Value (Signaling)") fxp<+/-,32,-16> 9.99982319171977e-11 ("Value (Signaling)") fxp<+/-,32,-16> 1.000000082740371e-09 ("Value (Signaling)")] -> w345
          frame 0, Default {
          }
          frame 1 {
          }
          frame 2 {
          }
          frame 3 {
          }
        }
        n147 = property on="ECG Beta" class="DigNum (strict)"("Val(Sgnl)"=w345) -> ()  [unwired: 2 in, 2 out]
      }
    }
  }
  n148 = while {
    tunnel: w45 -> [w359]
    tunnel: w43 -> [_]
    tunnel: w42 -> [_]
    tunnel: w34 -> [_]
    stop <- w358 stop-if-true
    n149 = Dequeue Element(queue=w359) -> (element=w357:i16[], error out=w358:errorcluster)  [unwired: 2 in, 2 out]
    n150 = case shown="No Error" w358 {
      tunnel: w357 -> [w376 _]
      frame No Error {
        n151 = local read "Trigger 2"() -> (w374:T3)
        n152 = property on="Invasive Blood Pressure" class="WFChart (strict)"() -> ("YScale.Ofst&Mult"=w364:T8)  [unwired: 2 in, 2 out]
        n153 = Cluster To Array(cluster="Plot Info") -> (array=w370:cluster{"Lead":T1, "Filter":bool}[])
        n154 = call "Parse Rx Data.vi"("Trigger"=w374, "Scale"=w364, "Plot Info"=w370, "Input Data"=w376) -> ("Pressures"=w366:i16[][], "Gradients"=w363:i16[][], "ECG Data"=→"ECG":i16[][], "Trigger"=→"Trigger":i16[][])  [unwired: 4 in]
        "Gradients" <- w363
        "Invasive Blood Pressure" <- w366
        n155 = Unbundle(w364) -> ("Offset"=w367:dbl, "Multiplier"=w369:dbl)
        n156 = Multiply(x=w369, y=w366) -> (x*y=w368:dbl[][])
        n157 = Add(x=w367, y=w368) -> (x+y=w365:dbl[][])
        n158 = Add Array Elements(numeric array=w363) -> (sum=w362:i16)
        n159 = Transpose 2D Array(2D array=w365) -> (transposed array=w371:dbl[][])
        n160 = Greater?(x=w362, y=i16 1000) -> (0:w360:bool)
        n161 = for {
          tunnel: w371 -> [w380] mode=indexing
          tunnel: [w377] -> _ mode=indexing
          n162 = Array Max & Min(array=w380) -> (max value=w379:dbl, min value=w378:dbl)  [unwired: 2 out]
          n163 = Bundle(w379, w378) -> (w377:cluster{dbl, dbl})  [unwired: 1 in]
        }
        n164 = local write "Active"(w360) -> ()
      }
      frame Error {
      }
    }
  }
  n165 = while {
    tunnel: w37 -> [w386]
    shift-right: [w385] -> _
    shift-left: -1 -> [w384]
    shift-right: [w382] -> _
    shift-left: _ -> [w381]
    tunnel: w3 -> [_]
    stop <- w383 stop-if-true
    n166 = event shown="[0] Timeout" {
      selector: _ -> [_ _ _]
      dyn-events: _ -> [_ _ _]
      timeout: w384 -> [_ _ _]
      tunnel: w386 -> [w393 _ _]
      tunnel: [w392 w430 _] -> w385
      tunnel: w384 -> [w392 _ _]
      tunnel: [w389 w427 errorcluster {"status"=TRUE, "code"=0, "source"=""} ("error IO")] -> w383
      tunnel: [w388 w429 w453] -> w382
      tunnel: w381 -> [w387 w428 w453]
      event Timeout {
        n167 = event-data() -> ()  [unwired: 1 in, 1 out]
        n168 = Dequeue Element(queue=w393, timeout in ms (-1)=10) -> (element=w394:i16[], timed out?=w390:bool, error out=w395:errorcluster)  [unwired: 1 in, 1 out]
        n169 = case shown="No Error" w395 {
          selector: w395 -> [w397 w423]
          tunnel: w394 -> [w400 _]
          tunnel: w390 -> [w399 _]
          tunnel: [w396 w423] -> w389
          tunnel: [w398 w422] -> w388
          tunnel: w387 -> [w398 w422]
          frame No Error {
            n170 = case shown="False" w399 {
              tunnel: w400 -> [w412 _]
              tunnel: w398 -> [w405 _]
              tunnel: w397 -> [w402 w421]
              tunnel: [w406 w421] -> w396
              frame False {
                n171 = Refnum to Path(1:w405) -> (0:w407:path)
                n172 = call <vilib>:"Check if File or Folder Exists.vi"("error in (no error)"=w402, "path"=w407) -> ("error out"=w403:errorcluster, "file or folder exists?"=w411:bool, "dup path"=w410:path)  [unwired: 7 in]
                n173 = case shown="False" w411 {
                  tunnel: w410 -> [w417 w420]
                  tunnel: [w416 w420] -> _
                  tunnel: w405 -> [w415 w419]
                  tunnel: [w415 w419] -> w404
                  tunnel: w403 -> [w414 w418]
                  tunnel: [w413 w418] -> w401
                  frame False {
                    n174 = Create Folder(path (use dialog)=w417, error in=w414) -> (created path=w416:path, error out=w413:errorcluster)  [unwired: 1 in, 1 out]
                  }
                  frame True {
                  }
                }
                n175 = call "Format Log Data.vi"("Array in"=w412) -> ("Array out"=w409:i16[][])  [unwired: 10 in]
                n176 = Write to Binary File(file (use dialog)=w404, data=w409, error in=w401, 5:TRUE ("prepend array or string size? (T)")) -> (error out=w406:errorcluster)  [unwired: 2 in, 2 out]
              }
              frame True {
              }
            }
          }
          frame Error {
          }
        }
      }
      event "Record Only Activity", "Record": Value Change {
        n177 = event-data() -> ()  [unwired: 1 in, 1 out]
        n178 = local read "Record Only Activity"() -> (w425:bool)
        n179 = local read "Record"() -> (w424:bool)
        n180 = local read "Active"() -> (w426:bool)
        n181 = case shown="True" w424 {
          tunnel: [-1 1] -> w430
          tunnel: [refnum<file> refnum ("refnum out") w443] -> w429
          tunnel: w428 -> [w432 _]
          tunnel: [w434 w442] -> w427
          tunnel: w426 -> [_ w440]
          tunnel: w425 -> [_ w439]
          frame False {
            n182 = Not A Number/Path/Refnum?(number/path/refnum=w432) -> (NaN/Path/Refnum?=w431:bool)
            n183 = case shown="False" w431 {
              tunnel: w432 -> [w437 _]
              tunnel: [w436 errorcluster {"status"=FALSE, "code"=0, "source"=""} ("error out")] -> w434
              frame False {
                n184 = Close File(refnum=w437) -> (error out=w436:errorcluster)  [unwired: 1 in, 1 out]
              }
              frame True {
              }
            }
          }
          frame True {
            n185 = Compound Arithmetic op=OR(w440, invert w439) -> (w441:bool)
            n186 = case shown="True" w441 {
              tunnel: [refnum<file> refnum ("refnum out") w448] -> w443
              tunnel: [errorcluster {"status"=FALSE, "code"=0, "source"=""} ("error out") w447] -> w442
              frame False {
              }
              frame True {
                n187 = local read "Path"() -> (w450:path)
                n188 = call "Create New File Name.vi"("File Extension"="bin", "Path"=w450) -> ("Path Out"=w451:path)
                n189 = Open/Create/Replace File(file path (use dialog)=w451, operation (0:open)=T9."open or create") -> (refnum out=w448:refnum<file>, error out=w447:errorcluster)  [unwired: 4 in, 1 out]
              }
            }
          }
        }
      }
      event "Global Stop": Mouse Up {
        n190 = event-data() -> ()  [unwired: 1 in, 3 out]
      }
    }
  }
  n191 = Release Queue(queue=w32) -> ()  [unwired: 2 in, 3 out]
  n192 = xnode ("Close FPGA VI Reference")("FPGA VI Reference In"=w48, "error in"=w50) -> ("error out"=w49:errorcluster)
  n193 = Release Queue(queue=w40) -> ()  [unwired: 2 in, 3 out]
  n194 = Release Queue(queue=w36) -> ()  [unwired: 2 in, 3 out]
  n195 = flat-sequence {
    tunnel: w49 -> [w456]
    frame #0 {
      n196 = local write "Global Stop"(FALSE ("Global Stop")) -> ()
      "error out" <- w456
    }
  }
